vi "OpenProjectWithCode.vi"   [LabVIEW 2020]
uses:
  <resource>/dialog/lvconfig.llb/LV Config Read String.vi
types:
  T1 = enum32{"Invalid", "Standard", "Closed", "Hidden", "Minimized", "Maximized"}
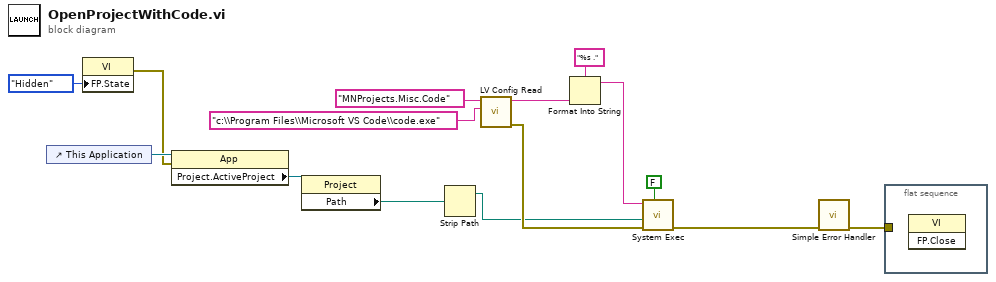
[diagram p0: block diagram]
diagram:
  n1 = control-ref of="This Application"() -> (w13:refnum<vi>)
  n2 = property class="VI"("FP.State"=T1."Hidden" ("Front Panel Window:State")) -> (error out=w1:errorcluster)  [unwired: 2 in, 1 out]
  n3 = property class="App"(reference=w13, error in=w1) -> ("Project.ActiveProject"=w12:refnum<vi>)  [unwired: 2 out]
  n4 = property class="Project"(reference=w12) -> ("Path"=w11:path)  [unwired: 1 in, 2 out]
  n5 = Strip Path(path=w11) -> (stripped path=w6:path)  [unwired: 1 out]
  n6 = call-poly <resource>:"LV Config Read.vi"("default value"="c:\\Program Files\\Microsoft VS Code\\code.exe" ("command line"), "key"="MNProjects.Misc.Code") -> ("error out"=w8:errorcluster, "value"=w4:string)  [unwired: 3 in, 1 out]
  n7 = Format Into String(format string="%s .", w4) -> (resulting string=w3:string)  [unwired: 2 in, 1 out]
  n8 = call <vilib>:"System Exec.vi"("wait until completion? (T)"=FALSE, "error in (no error)"=w8, "working directory"=w6, "command line"=w3) -> ("error out"=w14:errorcluster)  [unwired: 4 in, 3 out]
  n9 = call <vilib>:"Simple Error Handler.vi"("error in (no error)"=w14) -> ("error out"=w7:errorcluster)  [unwired: 4 in, 4 out]
  n10 = flat-sequence {
    tunnel: w7 -> [_]
    frame #0 {
      n11 = invoke class="VI" method="FP.Close"() -> ()  [unwired: 3 in, 3 out]
    }
  }
